vi "Write Temp Data HDF5 File.vi"(8 "Error In":errorcluster) -> (0 "Error Out":errorcluster)   [LabVIEW 2010]
uses:
  <vilib>/addons/h5labview2/file/H5F.lvlib
  <vilib>/addons/h5labview2/file/H5Fmode.ctl
  <vilib>/addons/h5labview2/dataset/H5Dwrite.llb/H5Dwrite.xnode
  <vilib>/addons/h5labview2/base/H5Equery.vi
  <vilib>/addons/h5labview2/base/lib_path.vi
panel:
  out "HDF5 File Path":path
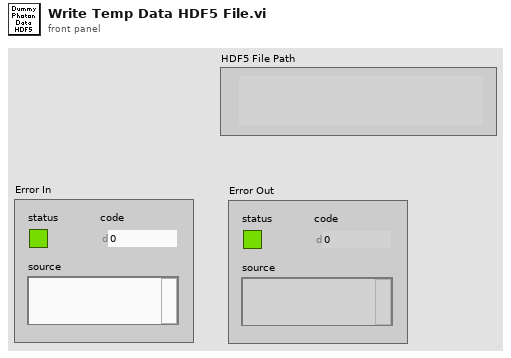
[diagram p1: front panel]
types:
  T1 = typedef "H5F.lvlib/H5Fmode.ctl" = enum16{"read-only", "read-write", "overwrite", "create new", "open or create"}
  T2 = typedef "hid_t.ctl" = i32
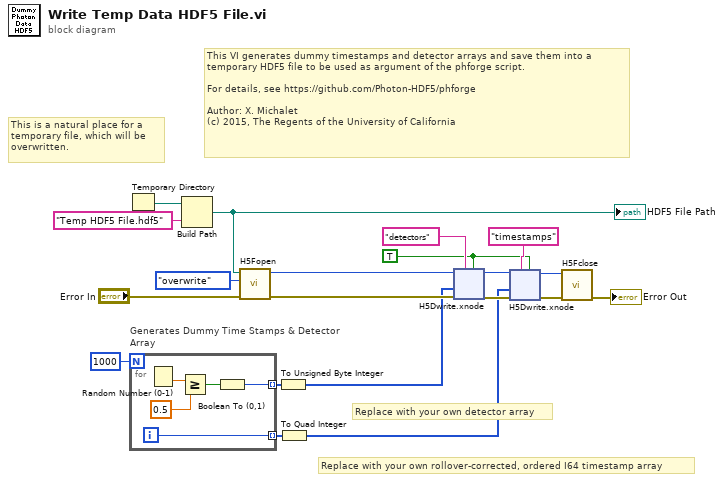
[diagram p0: block diagram]
diagram:
  w6 = TRUE ("replace? (F)")
  # "This is a natural place for a temporary file, which will be overwritten."
  # "Replace with your own detector array"
  # "Replace with your own rollover-corrected, ordered I64 timestamp array"
  # "This VI generates dummy timestamps and detector arrays and save them into a temporary HDF5 file to be used as argument of the phforge script.\n\nFor details, see https://github.com/Photon-HDF5/phforge\n\nAuthor: X. Michalet\n(c) 2015, The Regents of the University of California"
  n1 = Temporary Directory() -> (w18:path)
  n2 = for "Generates Dummy Time Stamps & Detector Array" {
    N: 1000 -> [_]
    tunnel: [w25] -> w5 mode=indexing
    tunnel: [w21] -> w11 mode=indexing
    i -> [w25]
    n3 = Random Number (0-1)() -> (number: 0 to 1=w24:dbl)
    n4 = Greater Or Equal?(x=w24, y=0.5) -> (x >= y?=w22:bool)
    n5 = Boolean To (0,1)(Boolean=w22) -> (0, 1=w21:i16)
  }
  n6 = Build Path(base path=w18, name or relative path="Temp HDF5 File.hdf5") -> (appended path=w16:path)
  "HDF5 File Path" <- w16
  n7 = call <vilib>:"H5Fopen.vi"("error in (no error)"="Error In", "mode (read-only)"=H5Fmode."overwrite", "path"=w16) -> ("error out"=w14:errorcluster, "ref out"=w13:T2)  [unwired: 7 in]
  n8 = To Unsigned Byte Integer(number=w11) -> (unsigned 8bit integer=w10:u8[])
  n9 = To Quad Integer(1:w5) -> (0:w4:i64[])
  n10 = xnode "H5Dwrite.xnode"("replace? (F)"=w6, "dataset name"="detectors" ("name"), "error in (no error)"=w14, "data"=w10, "ref in"=w13) -> ("error out"=w8:errorcluster, "ref out"=w9:i32)  [unwired: 2 in, 1 out]
  n11 = xnode "H5Dwrite.xnode"("replace? (F)"=w6, "dataset name"="timestamps", "error in (no error)"=w8, "data"=w4, "ref in"=w9) -> ("error out"=w3:errorcluster, "ref out"=w2:i32)  [unwired: 2 in, 1 out]
  n12 = call <vilib>:"H5Fclose.vi"("error in (no error)"=w3, "ref"=w2) -> ("error out"=→"Error Out":errorcluster)  [unwired: 9 in]
